vi "Compute Channel Indices.vi"(8 "error in (no error)":errorcluster, 9 "Next Index in":i32, 11 "Messages in":T1[](array[typedef]) {"Message Section Handle" format="%.0x"; "Parameter Channel Handles" format="%.0x"}) -> (0 "error out":errorcluster, 1 "Next Index out":i32, 2 "Channel Handles":T2[](array[typedef]) format="%.0x", 3 "Messages out":T1[](array[typedef]) {"Message Section Handle" format="%.0x"; "Parameter Channel Handles" format="%.0x"})   [LabVIEW 2020, in "AIM MIL-STD-1553 Engine.lvlib" / "Implementation.lvlib" / "Execution Unit.lvclass"]
uses:
  Execution Unit.lvclass
  <vilib>/NI VeriStand/Custom Device API/Custom Device Item Ref.ctl
  Custom Device/Compiled Message.ctl
  Shared/Direction.ctl
  Shared/Parameter Definition.ctl
  <vilib>/NI VeriStand/Custom Device API/Custom Device API.lvlib
  Custom Device/Custom Device.lvlib
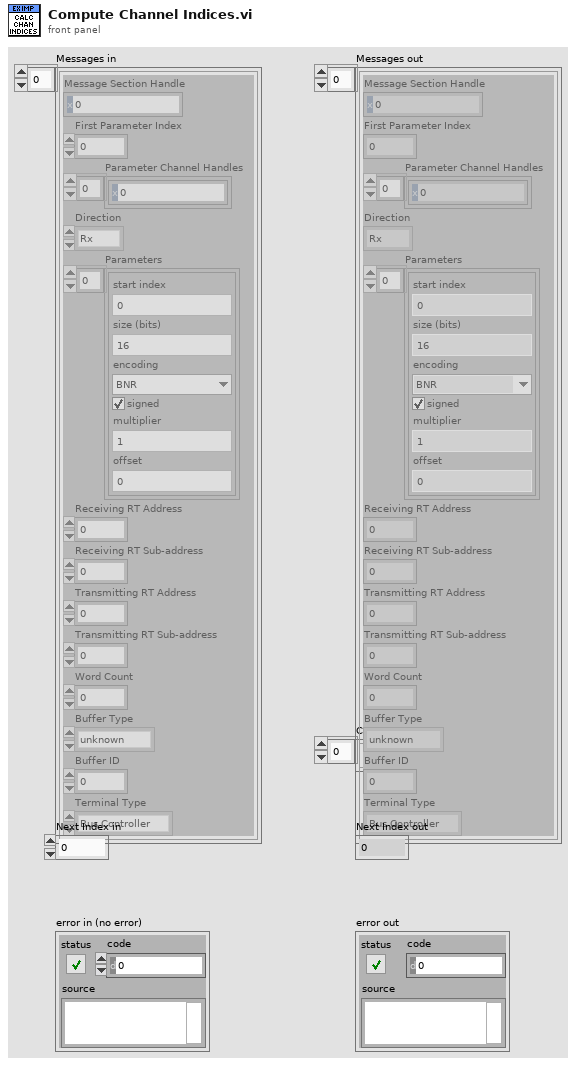
[diagram p1: front panel]
types:
  T1 = typedef "AIM MIL-STD-1553 Engine.lvlib/Custom Device.lvlib/Compiled Message.ctl" = cluster{"Message Section Handle":T2, "First Parameter Index":i32, "Parameter Channel Handles":T2[], "Direction":T3, "Parameters":T4[], "Receiving RT Address":u8, "Receiving RT Sub-address":u8, "Transmitting RT Address":u8, "Transmitting RT Sub-address":u8, "Word Count":u8, "Buffer Type":enum16{"unknown", "BC Message Buffer", "RT Message Buffer"}, "Buffer ID":u16, "Terminal Type":enum16{"Bus Controller", "Remote Terminal"}}
  T2 = typedef "Custom Device API.lvlib/Custom Device Item Ref.ctl" = u64
  T3 = typedef "Direction.ctl" = enum16{"Rx", "Tx"}
  T4 = typedef "Parameter Definition.ctl" = cluster{"start index":i32, "size (bits)":i32, "encoding":enum16{"BNR", "BCD", "Discrete"}, "signed":bool, "multiplier":dbl, "offset":dbl}
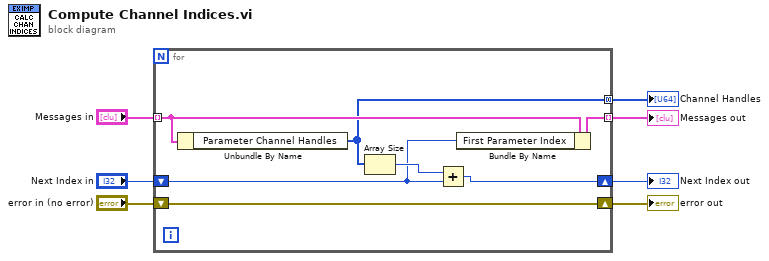
[diagram p0: block diagram]
diagram:
  n1 = for {
    tunnel: "Messages in" -> [w13] mode=indexing
    shift-right: [w14] -> w4
    shift-left: "error in (no error)" -> [w14]
    shift-right: [w11] -> w1
    shift-left: "Next Index in" -> [w10]
    tunnel: [w9] -> w6 mode=indexing
    tunnel: [w8] -> w7 mode=concatenating
    n2 = Unbundle By Name(w13) -> ("Parameter Channel Handles"=w8:T2[])
    n3 = Array Size(array=w8) -> (size(s)=w12:i32)
    n4 = Add(x=w12, y=w10) -> (x+y=w11:i32)
    n5 = Bundle By Name(cluster=w13, "First Parameter Index"=w10) -> (w9:T1)
  }
  "Channel Handles" <- w7
  "Messages out" <- w6
  "error out" <- w4
  "Next Index out" <- w1
